vi "dfd_PR Cosine-Modulated Augment Param.vi"(7 "M":i32=4, 9 "Initial phi":dbl[](array[numeric]), 10 "roll off":dbl=0.99, 11 "order":i32=39) -> (3 "Augmented phi":dbl[](array[numeric]), 5 "param":cluster{"M":i32, "Us":dbl[][], "roll off":dbl})   [LabVIEW 2017, in "NI_DigFilter_FilterBank.lvlib"]
uses:
  <vilib>/addons/Digital Filter Design/NI_DigFilter_FilterBank.lvlib
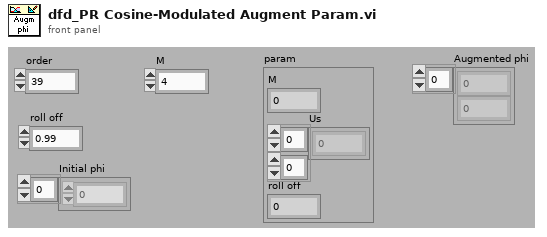
[diagram p1: front panel]
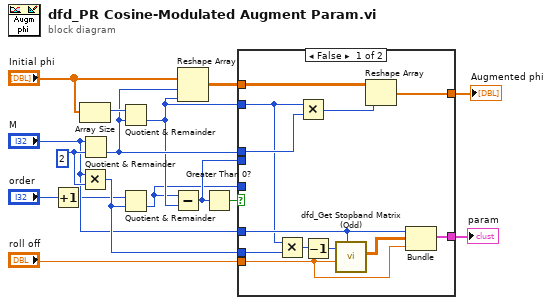
[diagram p0: block diagram]
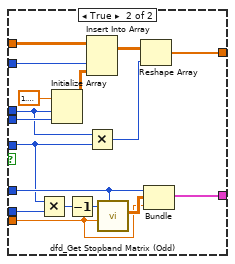
[diagram p2: hidden frame]
diagram:
  w14 = 2 ("y")
  n1 = Increment(x="order") -> (x+1=w3:i32)
  n2 = Array Size(array="Initial phi") -> (size(s)=w16:i32)
  n3 = Multiply(x="M", y=w14) -> (x*y=w8:i32)
  n4 = Quotient & Remainder(x="M", y=w14) -> (floor(x/y)=w11:i32)  [unwired: 1 out]
  n5 = Quotient & Remainder(x=w16, y=w11) -> (floor(x/y)=w5:i32)  [unwired: 1 out]
  n6 = Quotient & Remainder(x=w3, y=w8) -> (floor(x/y)=w2:i32)  [unwired: 1 out]
  n7 = Subtract(x=w2, y=w5) -> (x-y=w10:i32)
  n8 = Reshape Array("Initial phi", w11, w5) -> (w12:dbl[][])
  n9 = Greater Than 0?(x=w10) -> (x > 0?=w13:bool)
  n10 = case shown="False" w13 {
    tunnel: w12 -> [w28 w45]
    tunnel: w11 -> [w27 w39]
    tunnel: w10 -> [_ w43]
    tunnel: w5 -> [w20 w41]
    tunnel: w2 -> [_ w32]
    tunnel: [w25 w37] -> w9
    tunnel: w8 -> [w22 w34]
    tunnel: "M" -> [w23 w35]
    tunnel: "roll off" -> [w17 w29]
    tunnel: [w21 w33] -> w1
    frame False {
      n11 = Multiply(x=w20, y=w22) -> (x*y=w19:i32)
      n12 = Multiply(x=w20, y=w27) -> (x*y=w26:i32)
      n13 = Decrement(x=w19) -> (x-1=w18:i32)
      n14 = call <vilib>:"dfd_Get Stopband Matrix (Odd).vi"("number of bands"=w23, "roll off"=w17, "order"=w18) -> ("Us"=w24:dbl[][])  [unwired: 8 in]
      n15 = Reshape Array(w28, w26) -> (w25:dbl[])
      n16 = Bundle("M"=w23, "Us"=w24, "roll off"=w17) -> (w21:cluster{"M":i32, "Us":dbl[][], "roll off":dbl})  [unwired: 1 in]
    }
    frame True {
      n17 = Multiply(x=w32, y=w34) -> (x*y=w31:i32)
      n18 = Initialize Array(1.5707963267948966, w39, w43) -> (w42:dbl[][])
      n19 = Decrement(x=w31) -> (x-1=w30:i32)
      n20 = Insert Into Array(array=w45, index (col)=w41, new element=w42) -> (w40:dbl[][])  [unwired: 1 in]
      n21 = Multiply(x=w39, y=w32) -> (x*y=w38:i32)
      n22 = call <vilib>:"dfd_Get Stopband Matrix (Odd).vi"("number of bands"=w35, "roll off"=w29, "order"=w30) -> ("Us"=w36:dbl[][])  [unwired: 8 in]
      n23 = Reshape Array(w40, w38) -> (w37:dbl[])
      n24 = Bundle("M"=w35, "Us"=w36, "roll off"=w29) -> (w33:cluster{"M":i32, "Us":dbl[][], "roll off":dbl})  [unwired: 1 in]
    }
  }
  "Augmented phi" <- w9
  "param" <- w1
